vi "Download File.vi"(6 "Chunk size (kB)":i32=5120 min=5120, 8 "error in (no error)":errorcluster, 9 "Object Path":string, 10 "path to store downloaded file":path, 11 "Data.S3":refnum<class "LV-Data.S3.lvclass">) -> (0 "error out":errorcluster, 2 "file from jeff":path, 3 "Data.S3 out":refnum<class "LV-Data.S3.lvclass">)   [LabVIEW 2019, in "LV-Data.S3.lvclass"]
uses:
  LV-Data.S3.lvclass
  LV-Data.S3.lvclass/LV-Data.S3.ctl
  <vilib>/AWS Toolkit/S3/Bucket/Bucket.lvclass
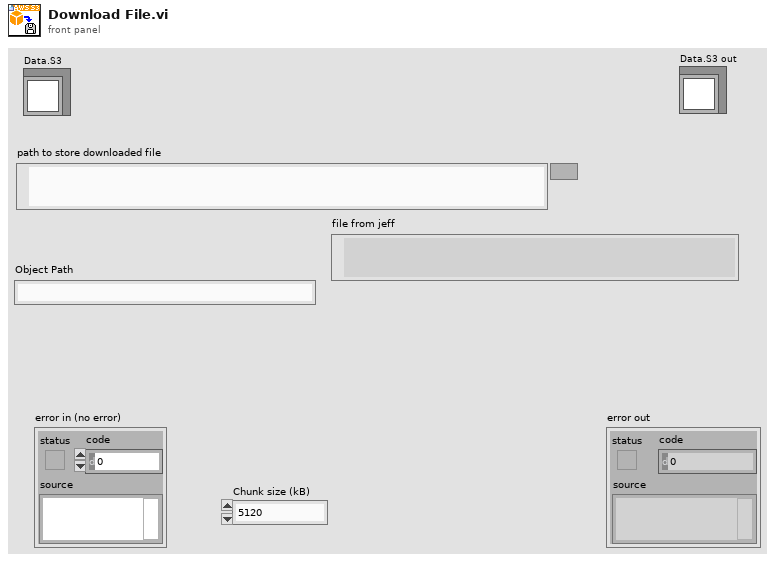
[diagram p1: front panel]
types:
  T1 = typedef "NI_AWS_Core.lvlib/HTTP Request.lvclass/AWS Credentials.ctl" = cluster{"Access Key":string, "Secret Key":string}
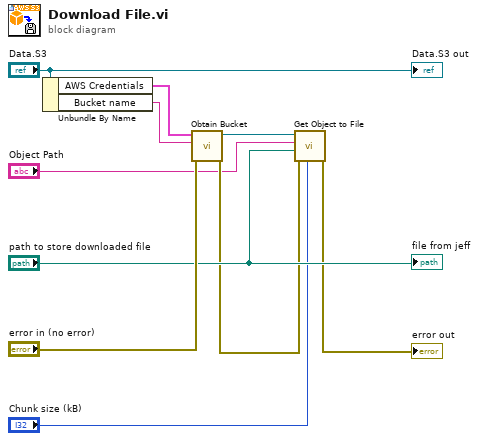
[diagram p0: block diagram]
diagram:
  n1 = Unbundle By Name("Data.S3") -> ("AWS Credentials"=w4:T1, "Bucket name"=w3:string)
  n2 = call <vilib>:"Obtain Bucket.vi"("error in (no error)"="error in (no error)", "Bucket name"=w3, "AWS Credentials"=w4) -> ("error out"=w8:errorcluster, "Bucket"=w5:refnum<class "Bucket.lvclass">)  [unwired: 7 in]
  n3 = call <vilib>:"Get Object to File.vi"("Chunk size (kB)"="Chunk size (kB)", "error in (no error)"=w8, "File"="path to store downloaded file", "Object Path"="Object Path", "Bucket in"=w5) -> ("error out"=→"error out":errorcluster)  [unwired: 5 in, 1 out]
  "file from jeff" <- "path to store downloaded file"
  "Data.S3 out" <- "Data.S3"
